vi "WriteToReport.vi"(8 "error in":errorcluster, 10 "Value":string, 11 "Header":T1="Low Pressure Initial") -> (0 "error out":errorcluster)   [LabVIEW 2018, in "S1.lvclass"]
uses:
  S1.lvclass
  Public Controls/ReportHeader.ctl
  Queue/Queue Data.ctl
  Queue/State.ctl
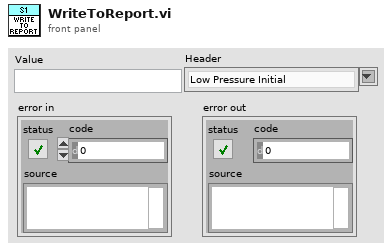
[diagram p1: front panel]
types:
  T1 = typedef "S1.lvclass/ReportHeader.ctl" = string
  T2 = typedef "S1.lvclass/Queue Data.ctl" = cluster{"State":T3, "Data":variant}
  T3 = typedef "S1.lvclass/State.ctl" = enum16{"Initialize", "SetConfig", "AckAlarm", "Alarm", "Idle", "LockLid", "LowPressure", "HighPressure", "Vent", "Abort", "Start", "CreateReports", "WriteToReport", "WritePressure", "Error", "Exit"}
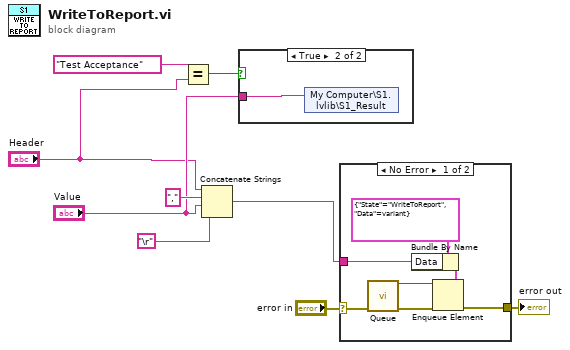
[diagram p0: block diagram]
diagram:
  n1 = Equal?(x=T1 "Test Acceptance" ("Header"), y="Header") -> (x = y?=w1:bool)
  n2 = Concatenate Strings("Header", "," ("string"), "Value", "\r") -> (w5:string)
  n3 = case shown="True" w1 {
    tunnel: "Value" -> [_ w10]
    frame False {
    }
    frame True {
      n4 = shared-variable "My Computer\\S1.lvlib\\S1_Result"(w10) -> ()  [unwired: 1 in, 1 out]
    }
  }
  n5 = case shown="No Error" "error in" {
    selector: "error in" -> [w17 w18]
    tunnel: [w14 w18] -> w9
    tunnel: w5 -> [w11 _]
    frame No Error {
      n6 = call "Queue.vi"("error in"=w17) -> ("error out"=w16:errorcluster, "queue out"=w15:refnum<queue>)  [unwired: 9 in]
      n7 = Bundle By Name(cluster=T2 {"State"=enum."WriteToReport", "Data"=variant} ("element"), "Data"=w11) -> (w12:T2)
      n8 = Enqueue Element(queue=w15, element=w12, error in (no error)=w16) -> (error out=w14:errorcluster)  [unwired: 1 in, 2 out]
    }
    frame Error {
    }
  }
  "error out" <- w9
